vi "show3.vi"(0 "Array":T1(array[cluster]), 3 "Multicolumn Listbox 2":refnum<vi>) -> (6 "max value":i32)   [LabVIEW 2014]
panel:
  out "Array 2":i32[](array[numeric])
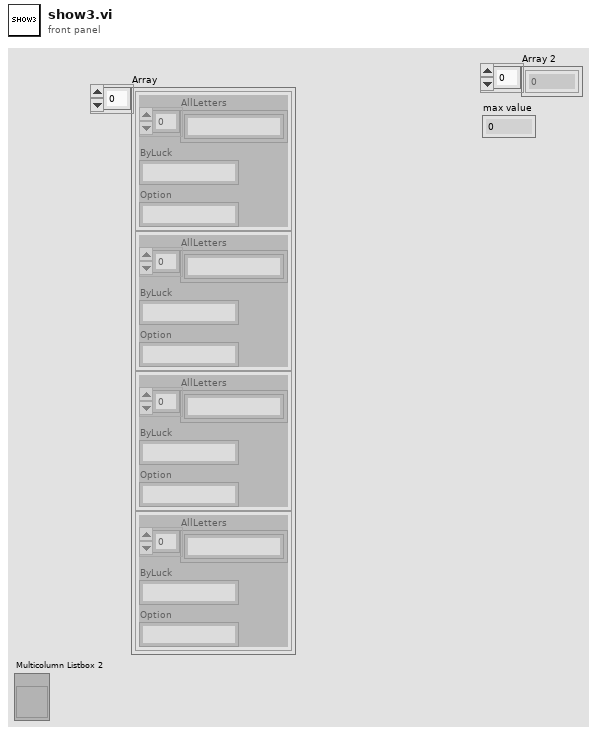
[diagram p1: front panel]
types:
  T1 = cluster{"AllLetters":string[], "ByLuck":string, "Option":string}[]
  T2 = cluster{"AllLetters":string[], "ByLuck":string, "Option":string}
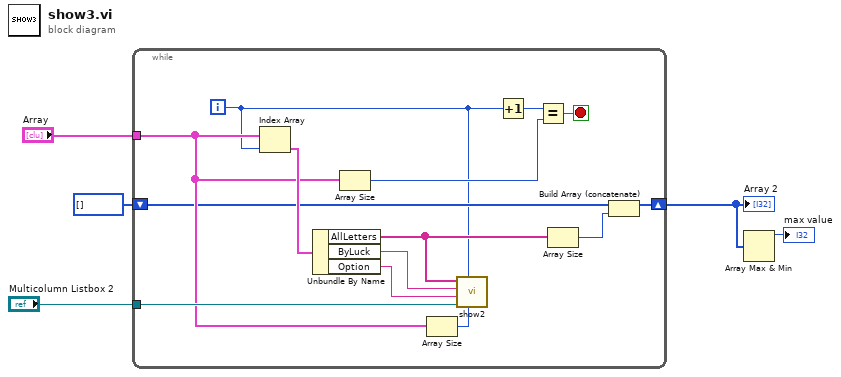
[diagram p0: block diagram]
diagram:
  n1 = while {
    tunnel: "Multicolumn Listbox 2" -> [w19]
    tunnel: "Array" -> [w12]
    shift-right: [w8] -> w2
    shift-left: i32[] [] -> [w7]
    i -> [w6]
    stop <- w14 stop-if-true
    n2 = Index Array(array=w12, index=w6) -> (element=w18:T2)
    n3 = Unbundle By Name(w18) -> ("AllLetters"=w10:string[], "ByLuck"=w16:string, "Option"=w17:string)
    n4 = Array Size(array=w12) -> (size(s)=w15:i32)
    n5 = Array Size(array=w12) -> (size(s)=w11:i32)
    n6 = call "show2.vi"("lines"=w11, "x"=w6, "reference"=w19, "OPTION"=w17, "first letter to find"=w16, "Array"=w10) -> ()  [unwired: 6 in]
    n7 = Increment(x=w6) -> (x+1=w13:i32)
    n8 = Equal?(x=w13, y=w15) -> (x = y?=w14:bool)
    n9 = Array Size(array=w10) -> (size(s)=w9:i32)
    n10 = Build Array (concatenate)(w7, w9) -> (w8:i32[])
  }
  "Array 2" <- w2
  n11 = Array Max & Min(array=w2) -> (max value=→"max value":i32)  [unwired: 3 out]
